vi "ServoControl.vi"(8 "error in (no error)":errorcluster, 10 "Channel Name":tag="B/PWM2", 11 "Position":dbl(slide)=1.5 scale=0.8..2.2 scale format="%#_3g") -> (0 "error out":errorcluster)   [LabVIEW 2017]
uses:
  <vilib>/Utility/error.llb/Error Cluster From Error Code.vi
  <vilib>/myRIO/Common/Instrument Driver Framework/myRIO v1.0/PWM/vis/myRIO v1.0 Write PWM.vi
  <vilib>/myRIO/Instrument Drivers/Onboard IO/PWM/PWM.lvlib
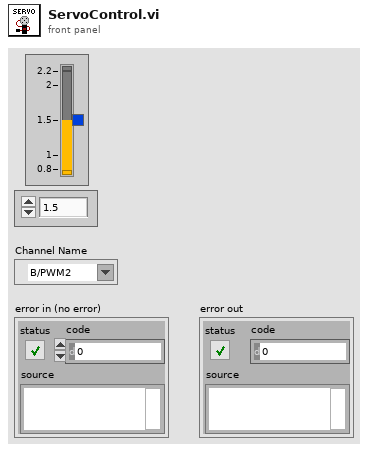
[diagram p1: front panel]
types:
  T1 = typedef "PWM.lvlib/PWM Reference.ctl" = cluster{"myRIO Reference":T2, "PWM Channels Enum":T6, "PWM Configuration":T7}
  T2 = typedef "myRIO Generic Hardware Reference.ctl" = cluster{"myRIO Model":T3, "myRIO Hardware Reference":T4}
  T3 = typedef "Hardware Version Enum.ctl" = enum16{"Unknown", "myRIO-1900", "myRIO-1950", "roboRIO", "NI ELVIS RIO CM"}
  T4 = typedef "myRIO v1.0 Reference.ctl" = cluster{"Generic FPGA Reference":T5, "Allow multiple opens":bool}
  T5 = typedef "Generic FPGA Reference.ctl" = refnum<k20>
  T6 = typedef "PWM Channels Enum.ctl" = enum16{"Not Connected", "C/PWM0", "C/PWM1", "A/PWM0", "A/PWM1", "A/PWM2", "B/PWM0", "B/PWM1", "B/PWM2", "PWM/PWM0", "PWM/PWM1", "PWM/PWM2", "PWM/PWM3", "PWM/PWM4", "PWM/PWM5", "PWM/PWM6", "PWM/PWM7", "PWM/PWM8", "PWM/PWM9"}
  T7 = typedef "PWM.lvlib/PWM Configuration.ctl" = cluster{"Frequency":dbl, "Duty Cycle":dbl}
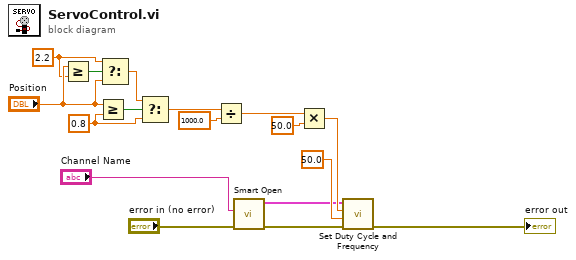
[diagram p0: block diagram]
diagram:
  w14 = 0.8 ("y")
  w12 = 2.2 ("y")
  n1 = Greater Or Equal?(x="Position", y=w12) -> (x >= y?=w11:bool)
  n2 = Greater Or Equal?(x="Position", y=w14) -> (x >= y?=w16:bool)
  n3 = Select(t=w12, s=w11, f="Position") -> (s? t:f=w15:dbl)
  n4 = Select(t=w15, s=w16, f=w14) -> (s? t:f=w17:dbl)
  n5 = Divide(x=w17, y=1000.0) -> (x/y=w2:dbl)
  n6 = call <vilib>:"Smart Open.vi"("error in (no error)"="error in (no error)", "Channel Name"="Channel Name") -> ("error out"=w6:errorcluster, "PWM Ref Out"=w5:T1)  [unwired: 8 in]
  n7 = Multiply(x=w2, y=50.0) -> (x*y=w9:dbl)
  n8 = call <vilib>:"Set Duty Cycle and Frequency.vi"("error in (no error)"=w6, "Frequency [Hz]"=50.0 ("Frequency (Hz)"), "Duty Cycle"=w9, "PWM Ref In"=w5) -> ("error out"=→"error out":errorcluster)  [unwired: 5 in, 1 out]
